vi "projekt.vi"() -> ()   [LabVIEW 2023]
doc: "Use this template to build a standard state machine design pattern. Each state executes code and determines which state to transition to. Contrast this design pattern with the User Interface Event Handler pattern, in which code executes in response to user actions. Contrast this design pattern also with the Queued Message Handler pattern, in which each message handling code can queue zero or more new messages.\nNote: This template does not contain the most recent programming guidelines recommended by National Instruments. For a complete, project-based implementation of the Standard State Machine pattern, use the Create Project dialog box instead of this template."
uses:
  projekt_stany.ctl
  <vilib>/DAQmx/read.llb/DAQmx Read (Digital 1D Bool 1Chan 1Samp).vi
  <vilib>/DAQmx/create/channels.llb/DAQmx Create Channel (DI-Digital Input).vi
  <vilib>/DAQmx/miscellaneous.llb/DAQmx Fill In Error Info.vi
panel:
  in  "Wyczysc":bool
  out "String 9":string
  out "String 8":string
  out "String 7":string
  out "String 6":string
  out "String 5":string
  out "String 4":string
  out "String 3":string
  out "String 2":string
  out "String":string
  out "Nastepny Gracz":string
  in  "Wybierz Kto zaczyna":bool
  out "Wynik":string
  in  "Stop":bool
  out "Kolumna":dbl
  out "Wiersz":dbl
  # "INSTRUKCJA GRY:"
  # "Aby wyczysc plansze, nalezy kliknac przycisk WYCZYSC na panelu glownym\noraz zatwierdzic CZERWONYM przyciskiem."
  # "Mozna wybrac kolejnosc czy O ma byc pierwsze czy moze X:\n - Jezeli przycisk jest wlaczony to zaczyna gracz X\n - Jezeli przycisk jest wylaczony to zaczyna gracz O\n\nJednak kolejnosc musi byc wybrana przed zaczeciem gry."
  # "Aby wybrac pole w którym ma byc wstawiony symbol nalezy wybrac kolumne oraz wiersz  (1 - 3) uzywajac przyciskow na urzadzeniu, aby dowiedziec sie za co opowiadaja przyciski przejdz do sekcji \"INSTRUKCJA DO PRZYCISKÓW\""
  # "INSTRUKCJA DO PRZYCISKÓW:"
  # "- Do wyboru wiersza sluzy przycisk ZIELONY\n - Do wyboru kolumny sluzy przycisk NIEBIESKI\n - Do zatwierdzenia swojego wyboru sluzy przycisk CZERWONY"
  # "SCHEMAT WYBORU POLA:"
  # "SCIAGAWKA PRZY WYBIERANIU POLA:"
  # "[ WIERSZ, KOLUMNA ]"
  # "[ 1, 1 ]  [ 1, 2 ]  [ 1, 3 ]\n[ 2, 1 ]  [ 2, 2 ]  [ 2, 3 ]\n[ 3, 1 ]  [ 3, 2 ]  [ 3, 3 ]"
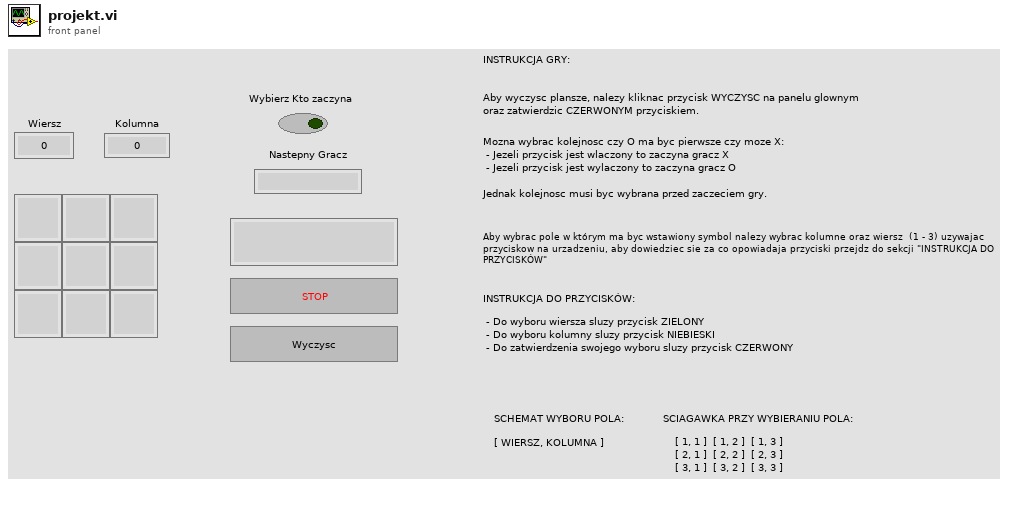
[diagram p1: front panel]
types:
  T1 = typedef "projekt_stany.ctl" = enum16{"Czysc", "Zapisz", "Wpisz", "Sprawdz", "Czytaj", "Initialize", "Stop"}
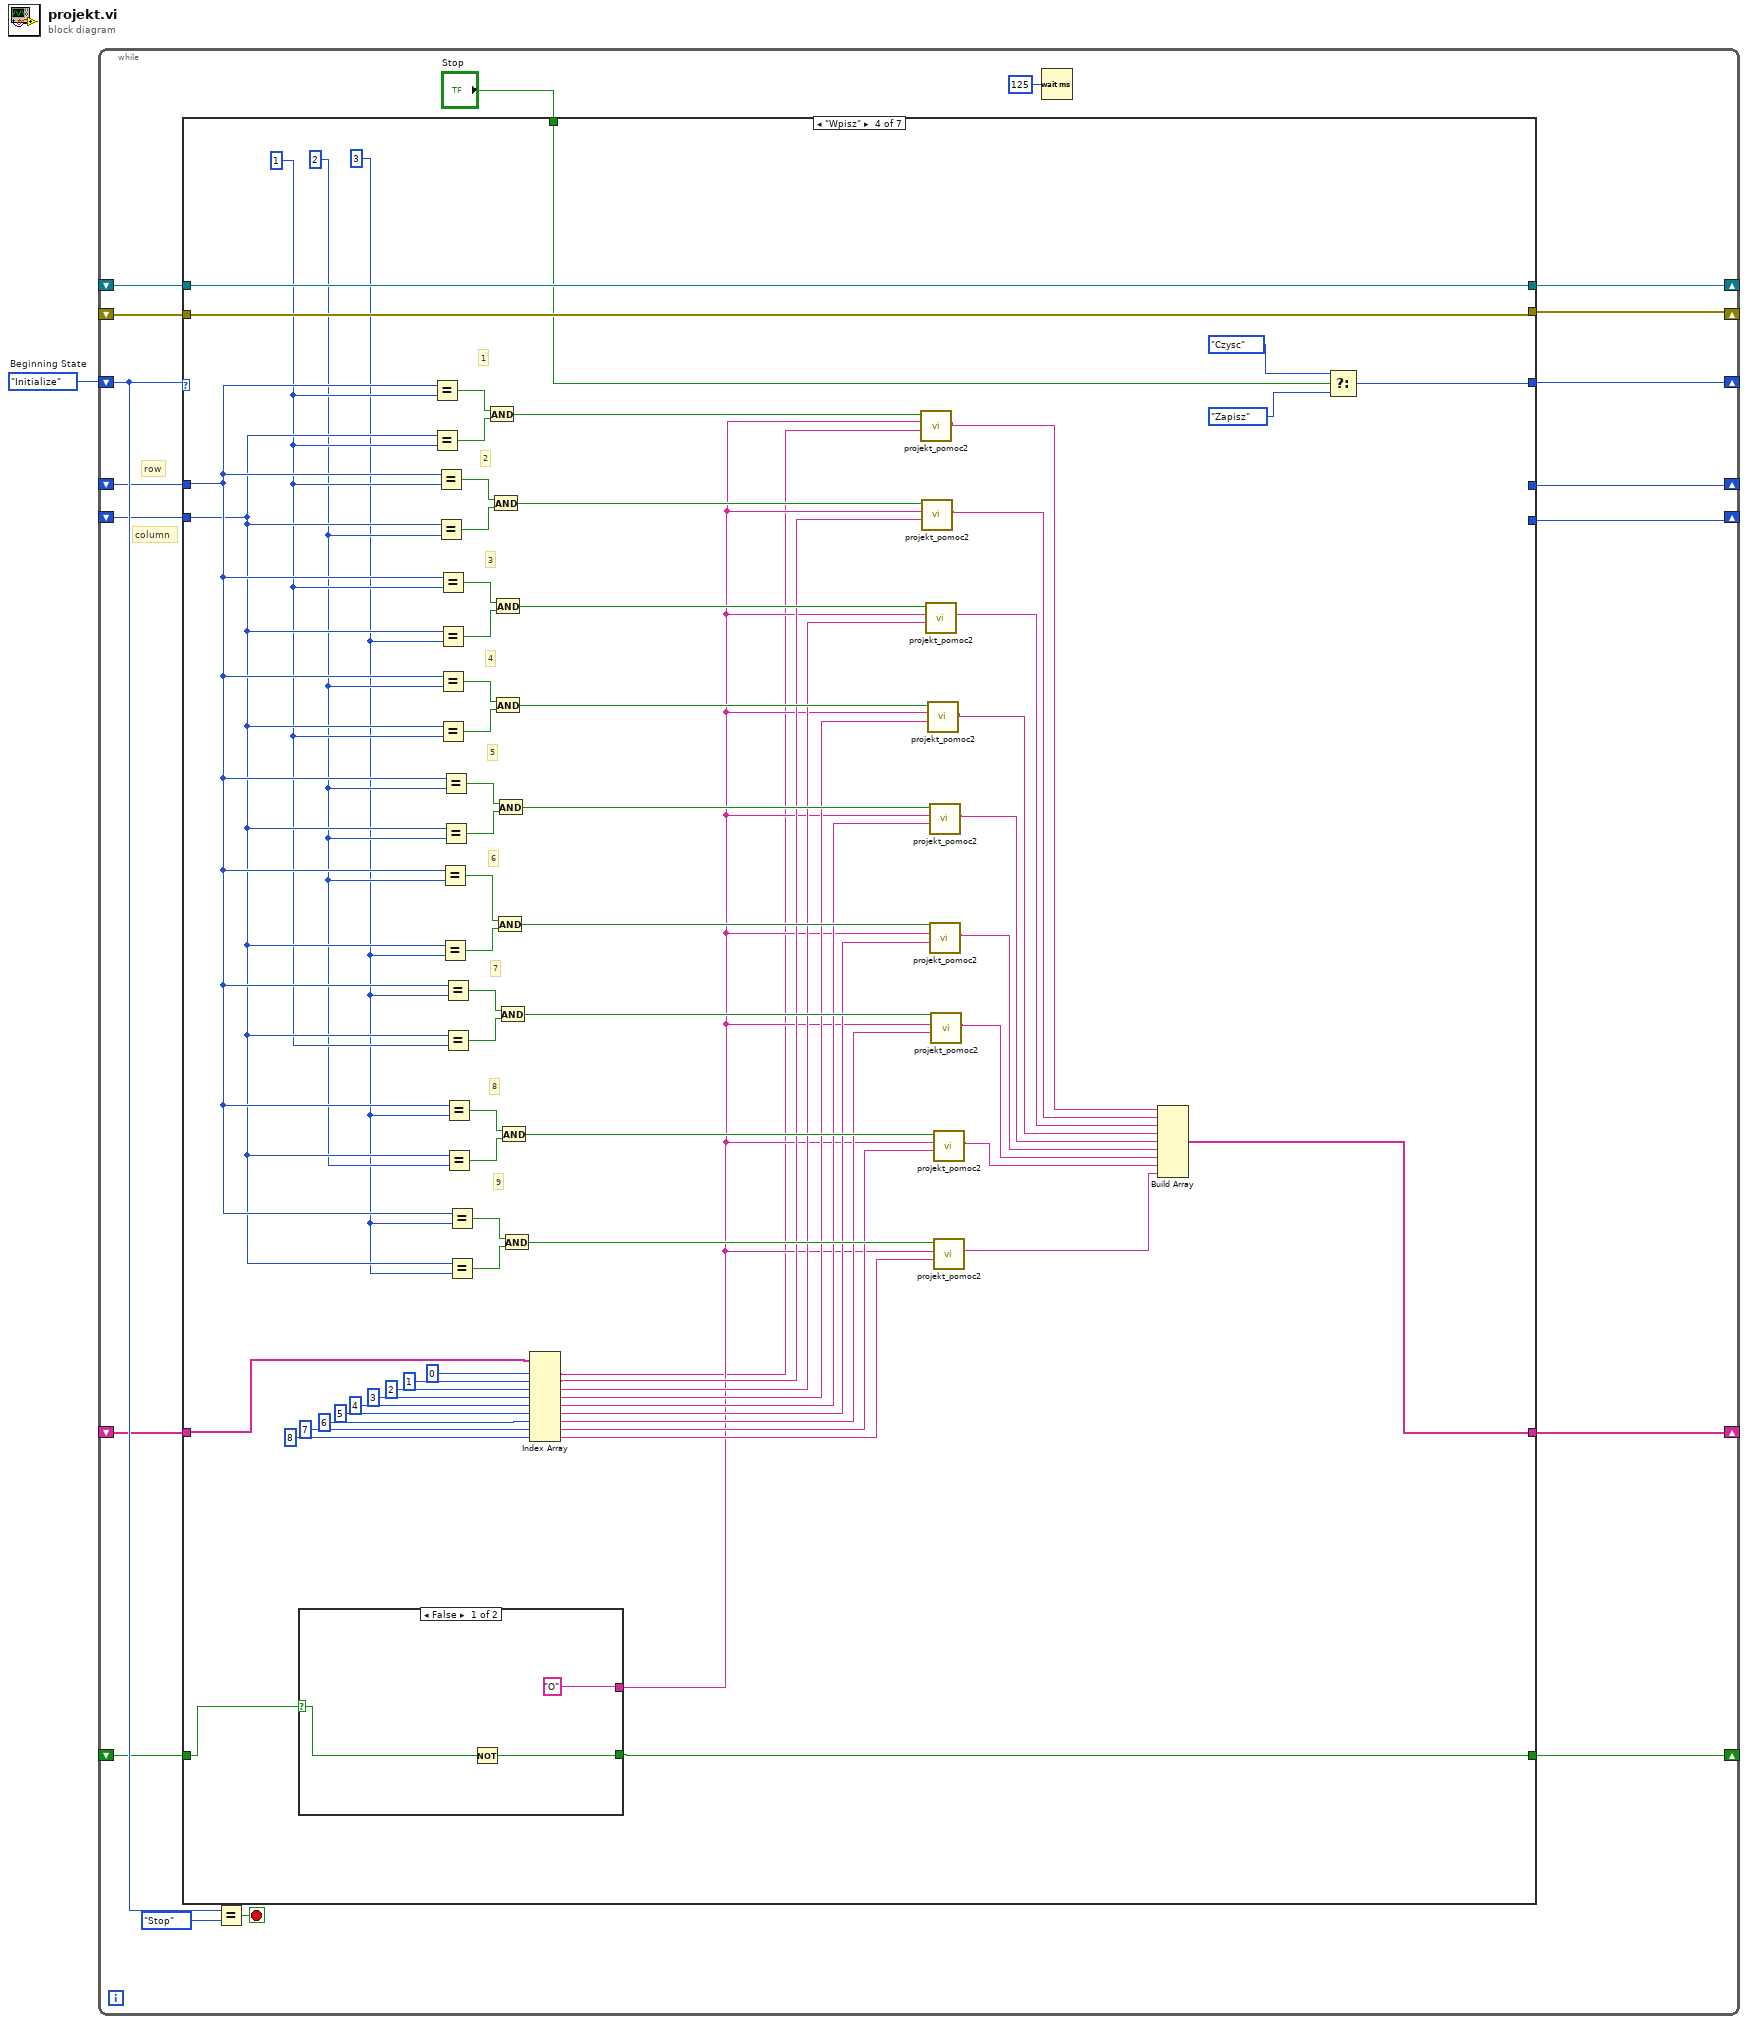
[diagram p0: block diagram]
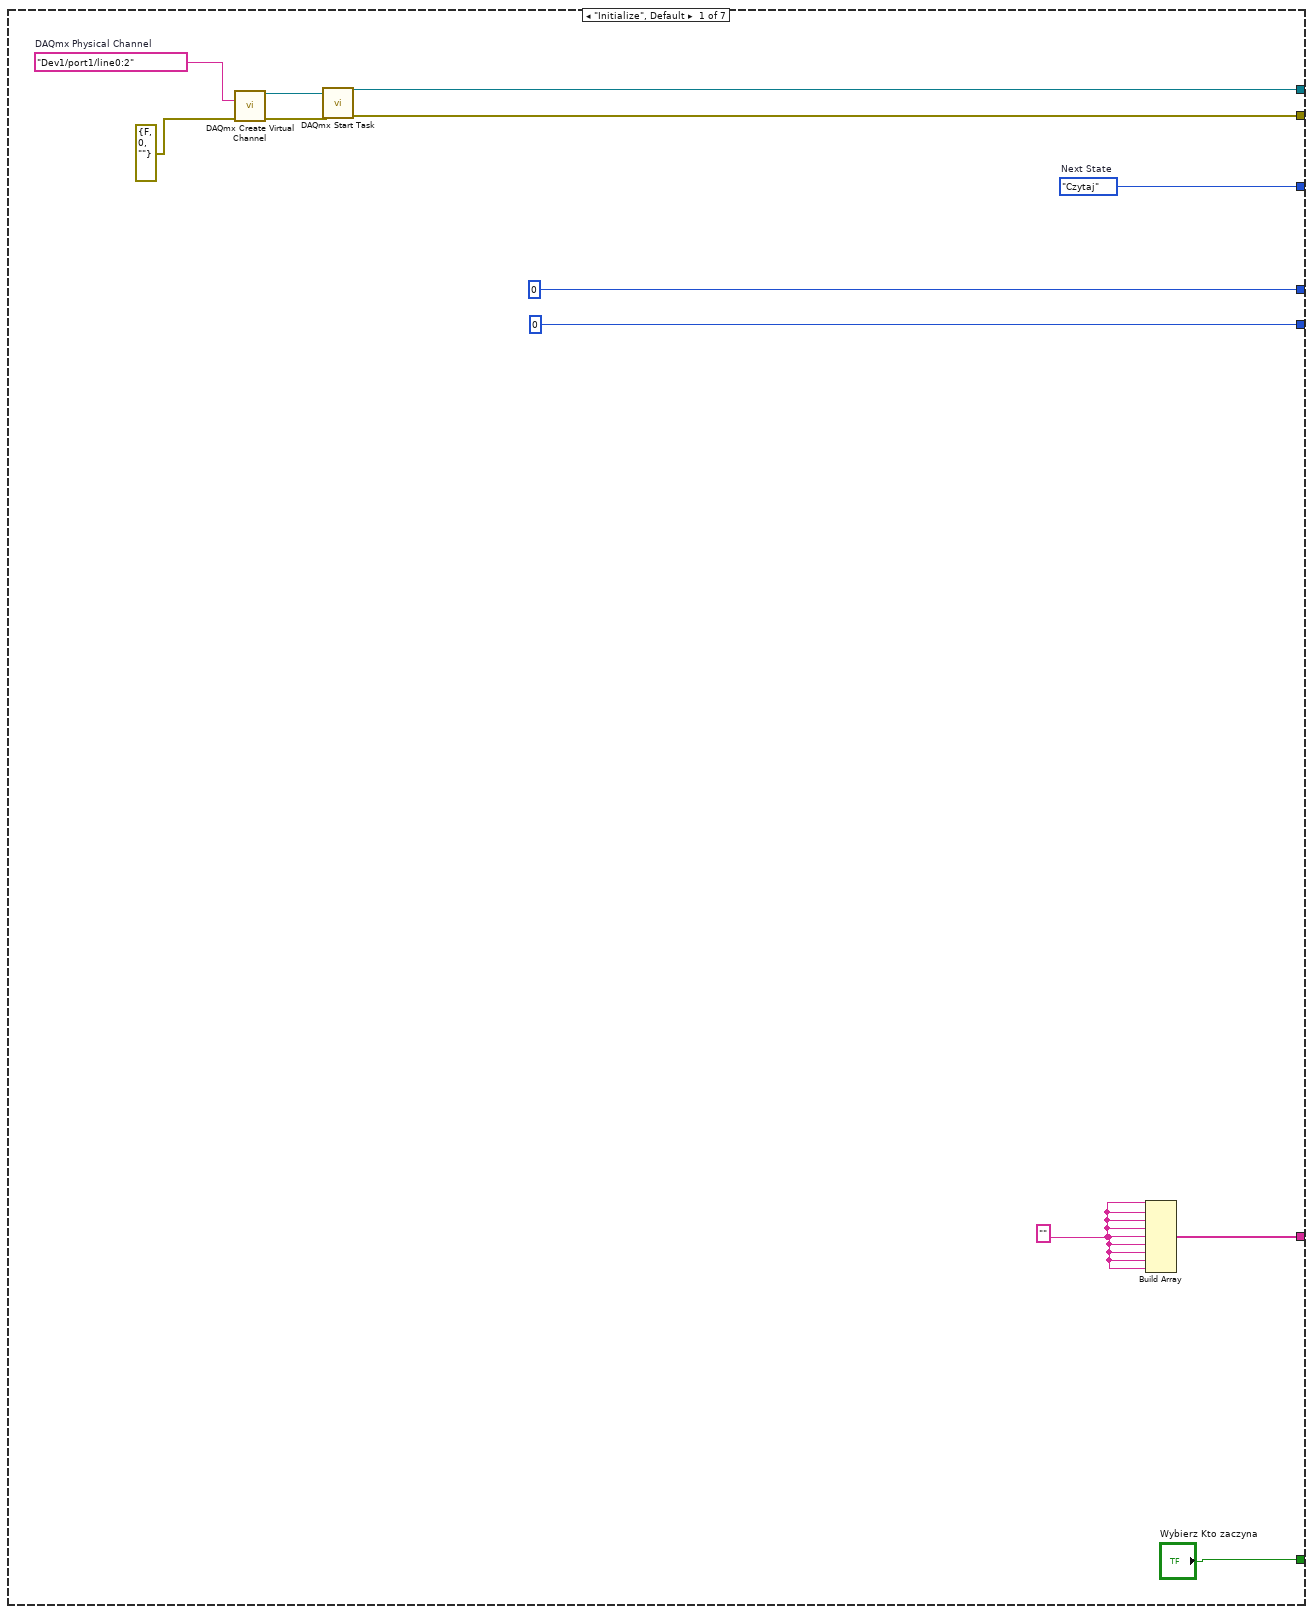
[diagram p2: hidden frame]
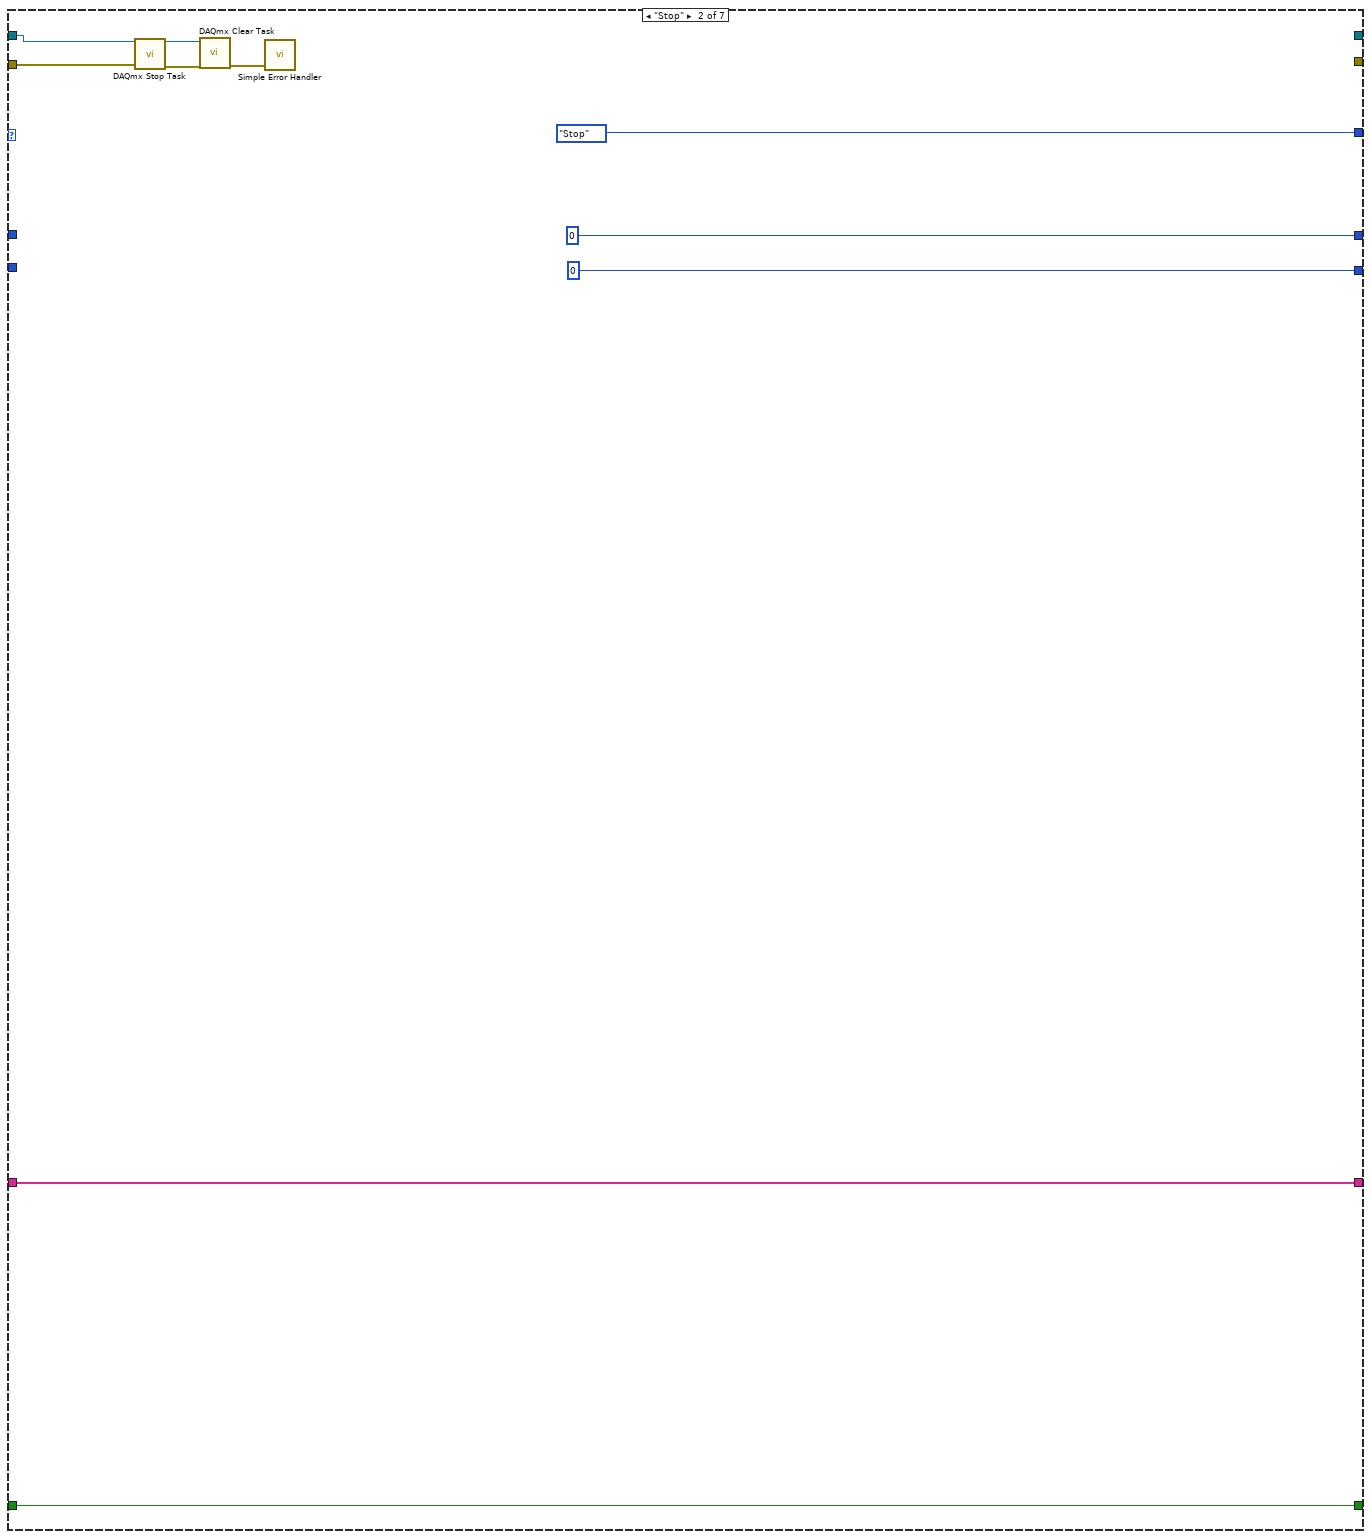
[diagram p3: hidden frame]
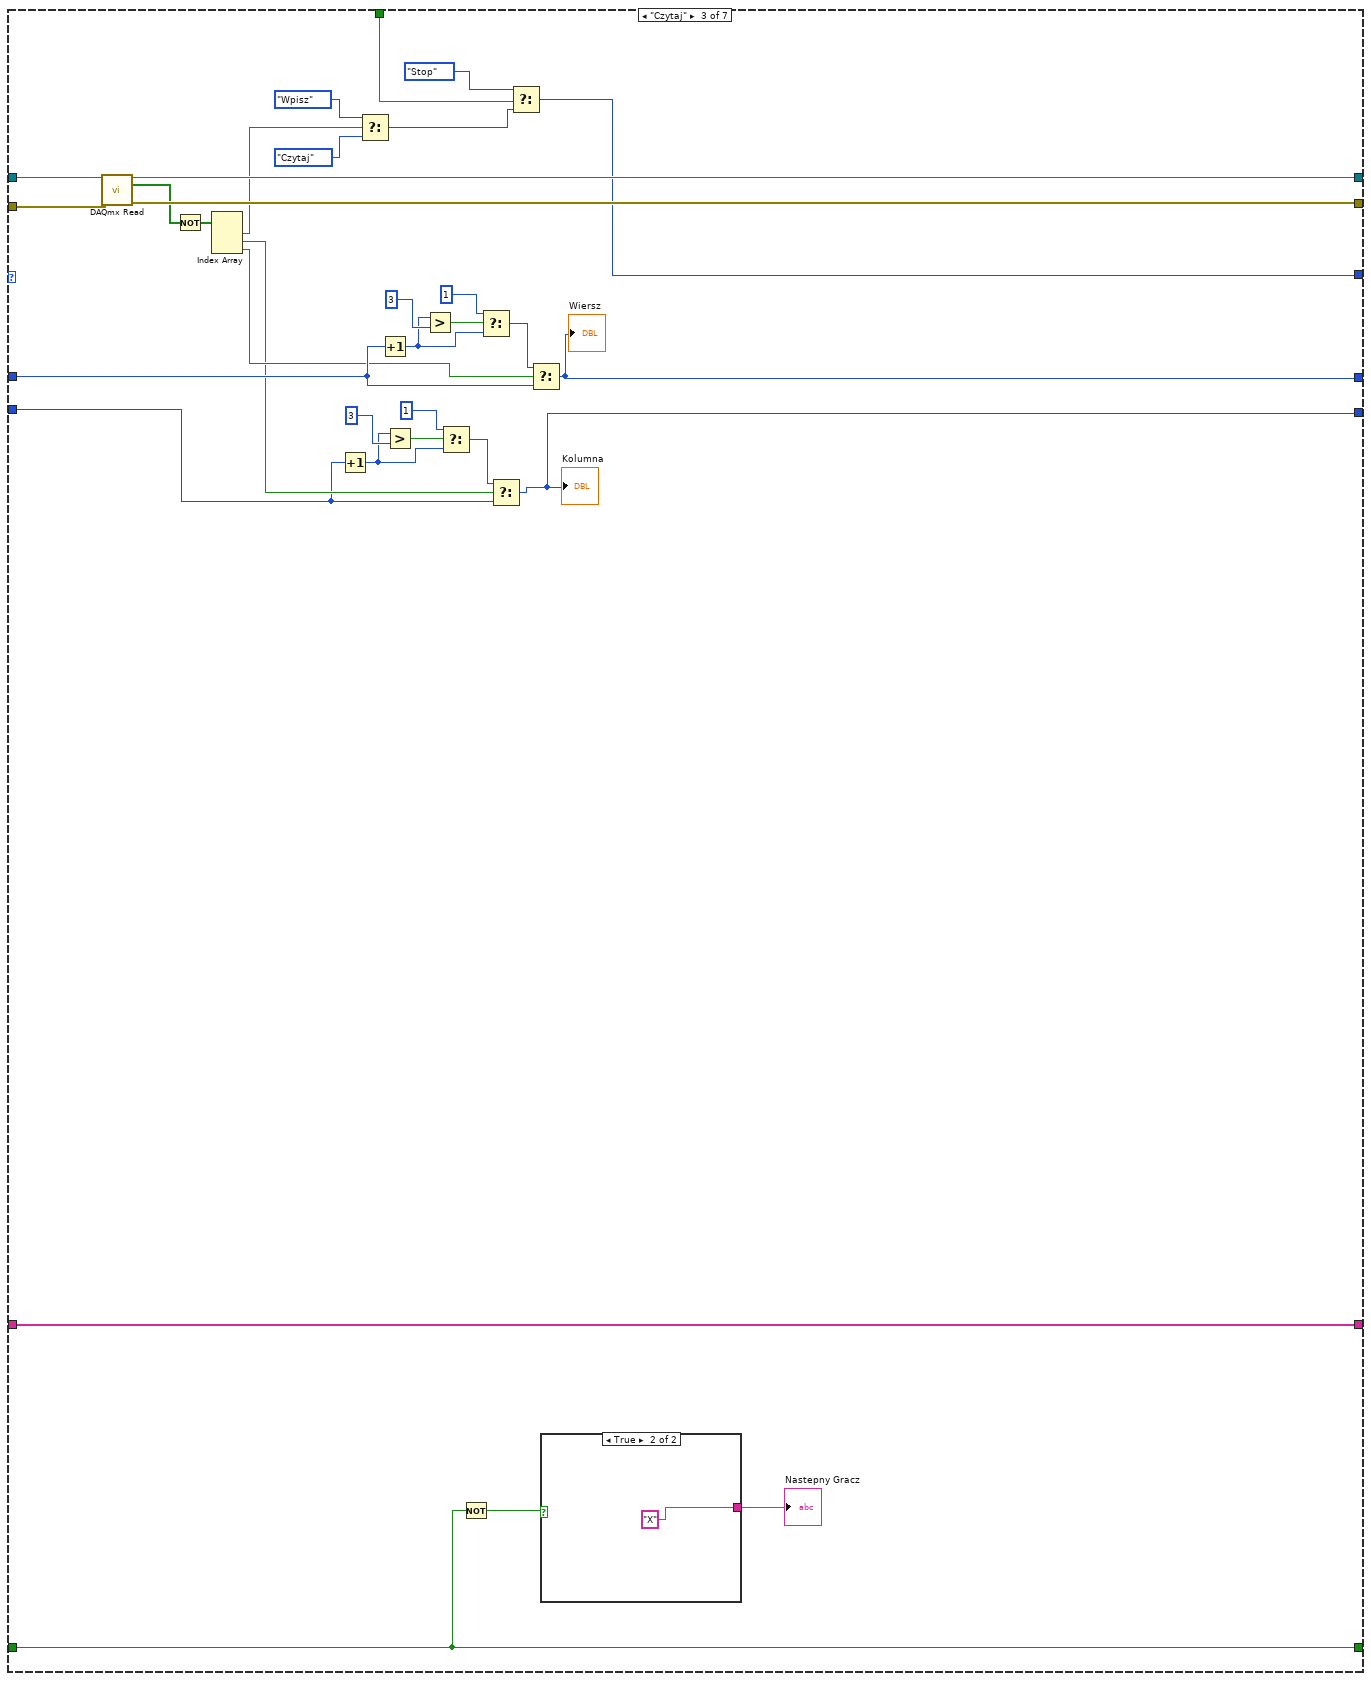
[diagram p4: hidden frame]
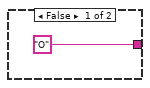
[diagram p5: hidden frame]
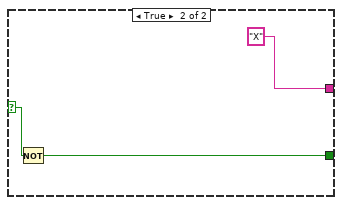
[diagram p6: hidden frame]
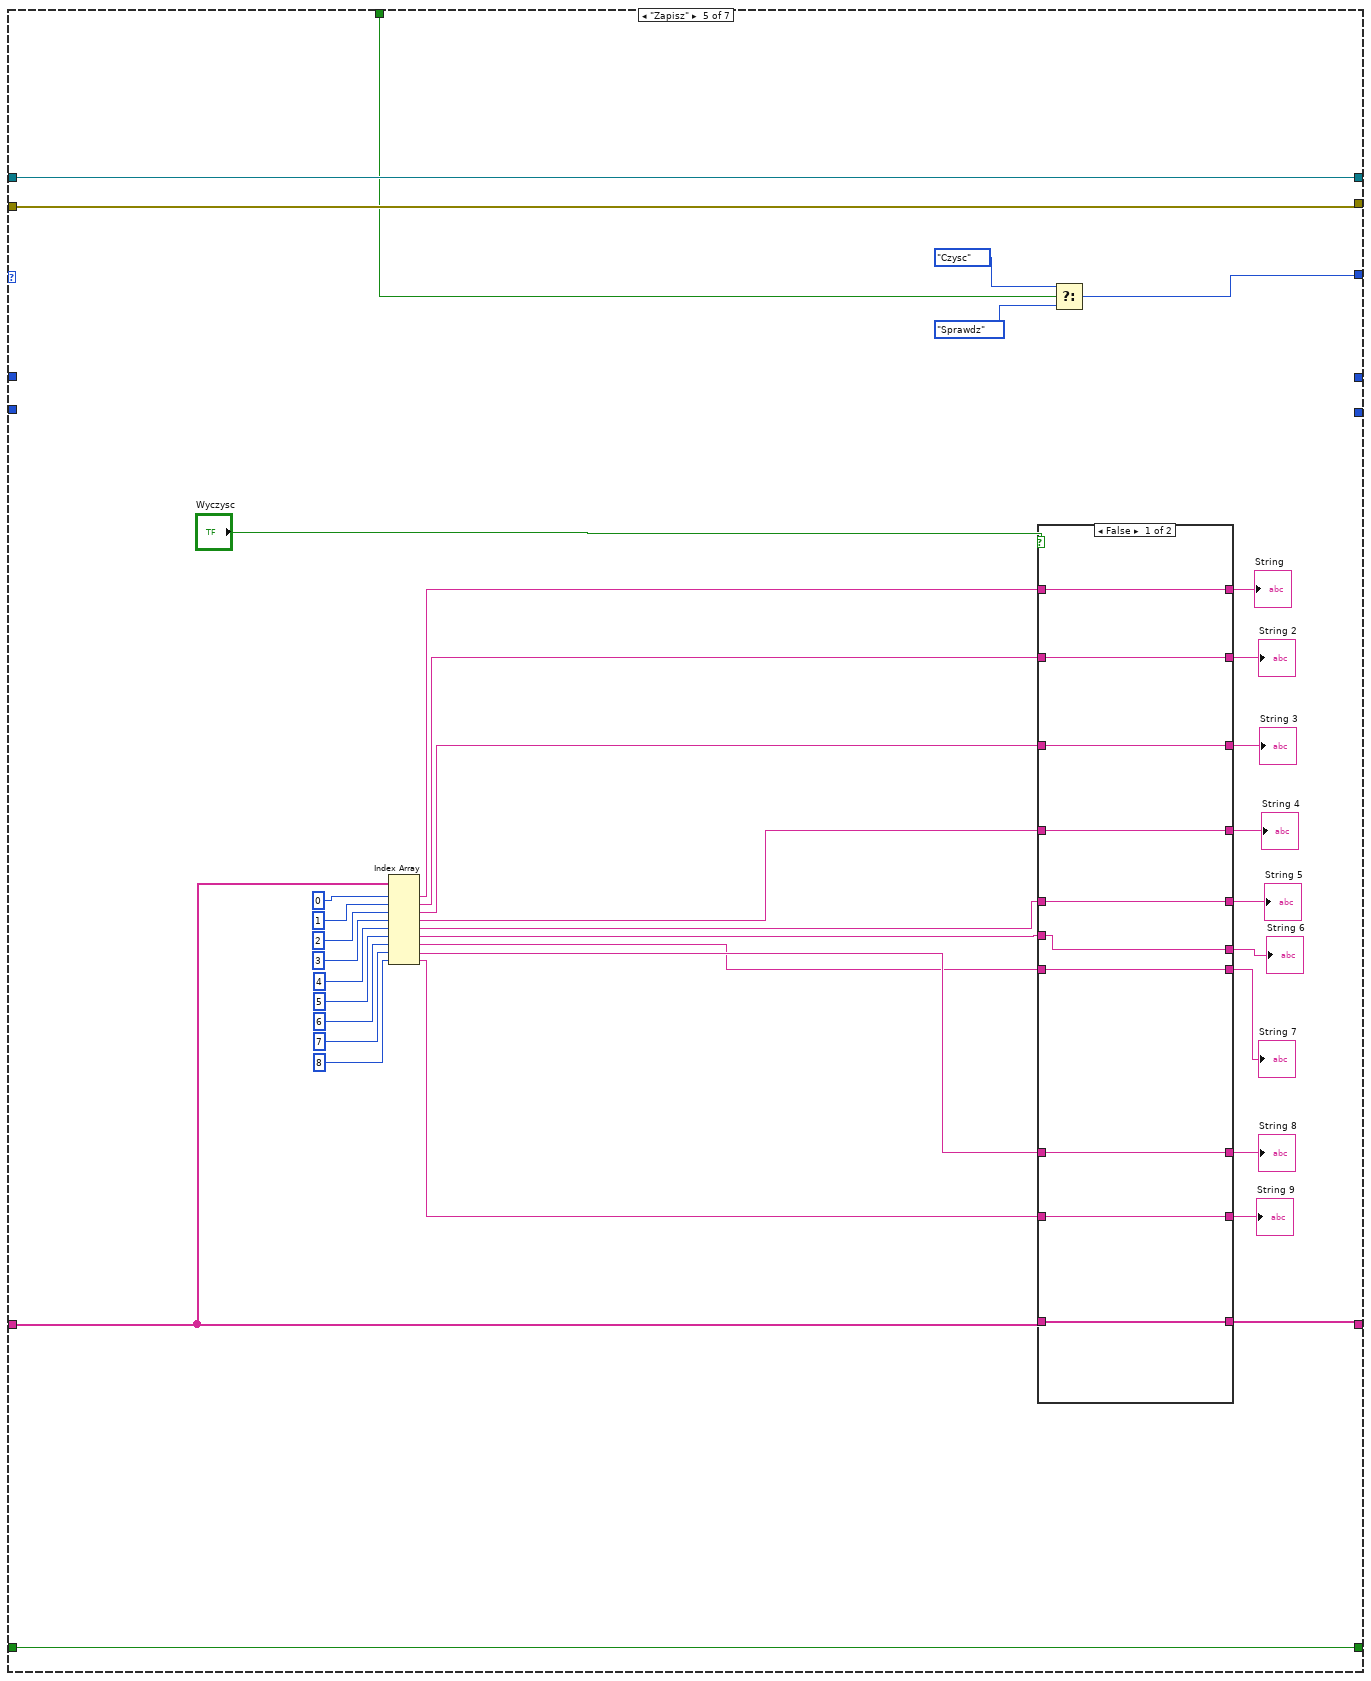
[diagram p7: hidden frame]
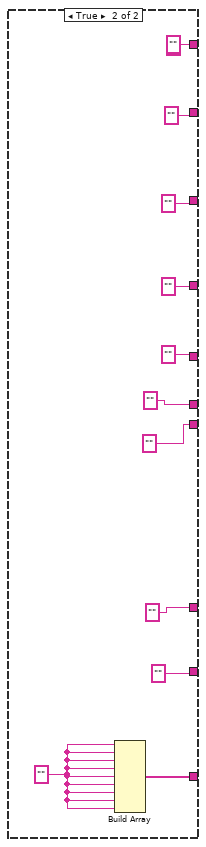
[diagram p8: hidden frame]
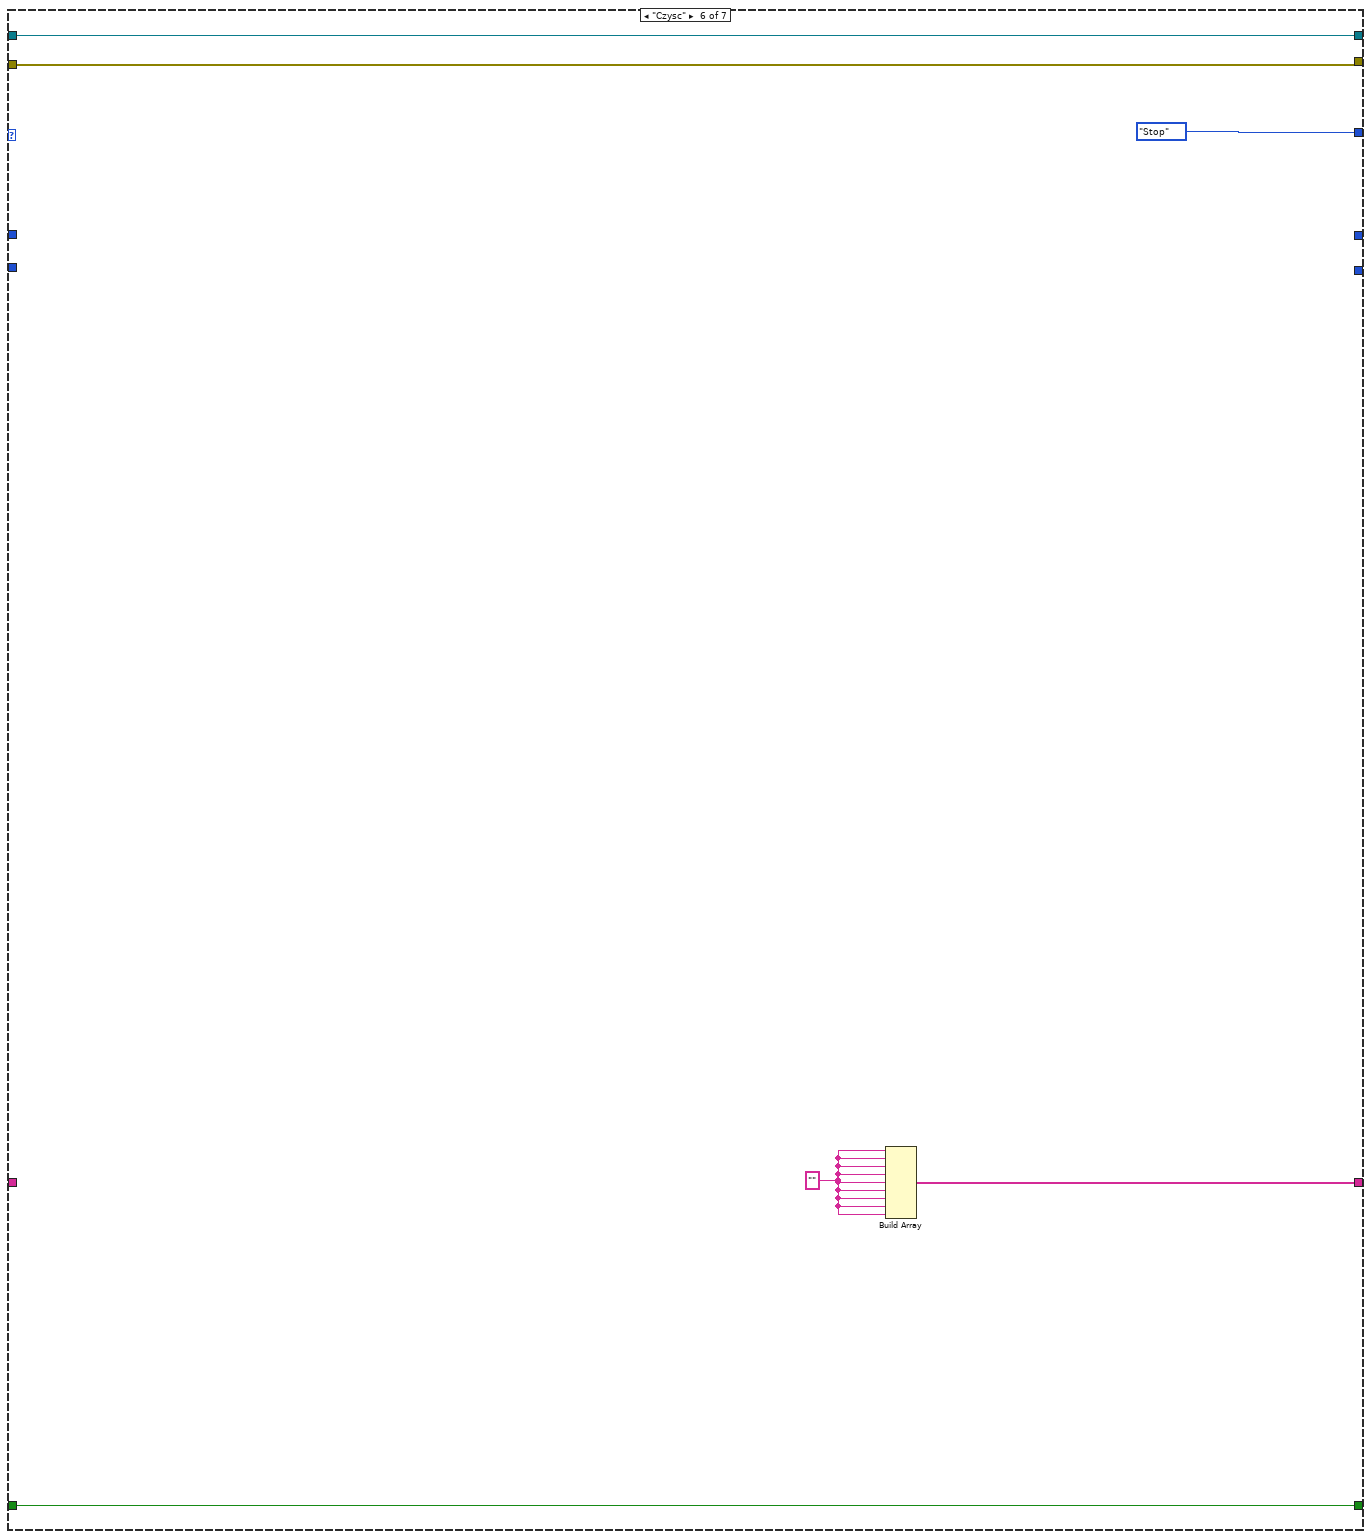
[diagram p9: hidden frame]
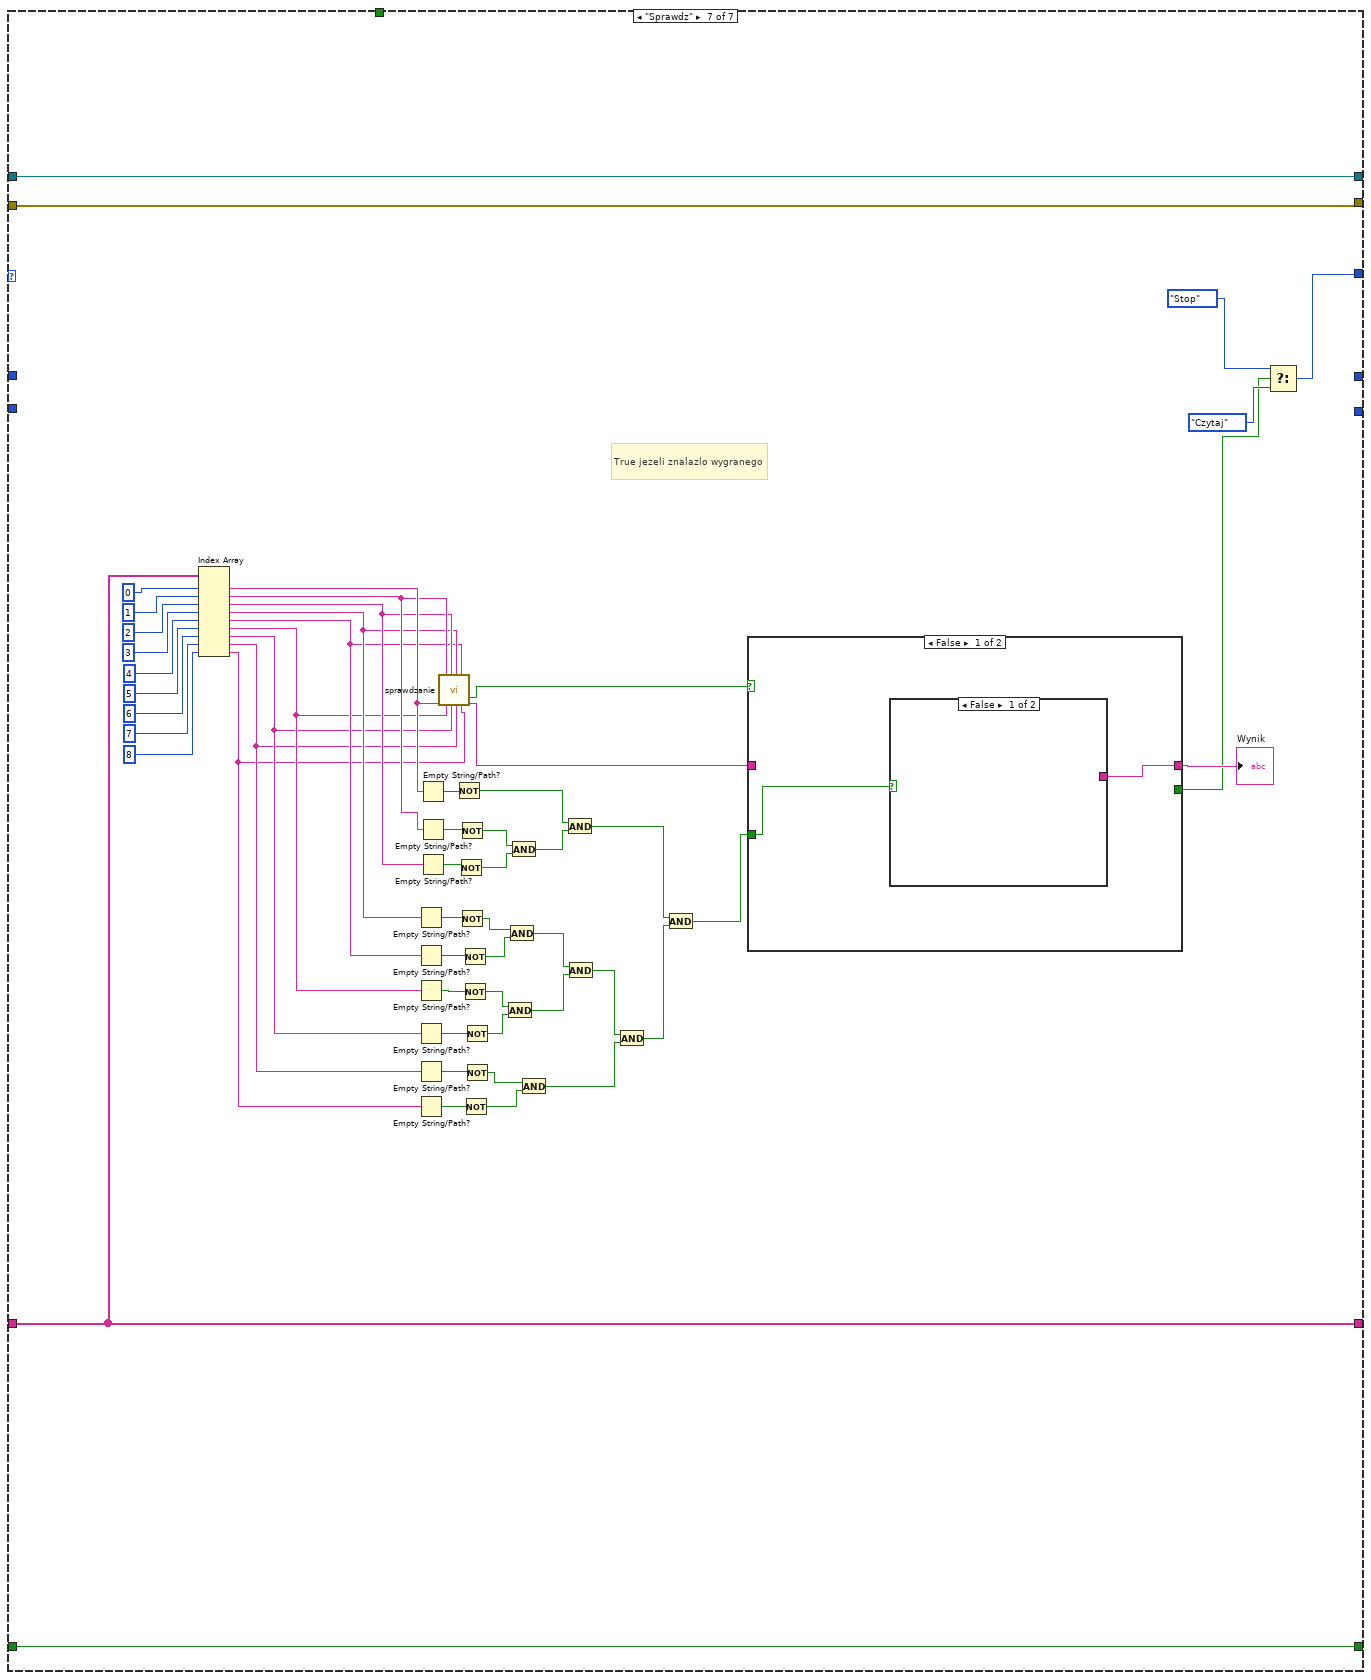
[diagram p10: hidden frame]
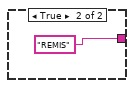
[diagram p11: hidden frame]
diagram:
  w1 = projekt_stany."Initialize"  # Beginning State
  n1 = while {
    shift-right: [w16] -> _
    shift-left: w1 -> [w17]
    shift-right: [w14] -> _
    shift-left: _ -> [w12]
    shift-right: [w13] -> _
    shift-left: _ -> [w11]
    shift-right: [w10] -> _
    shift-left: _ -> [w7]
    shift-right: [w9] -> _
    shift-left: _ -> [w8]
    shift-right: [w5] -> _
    shift-left: _ -> [w4]
    shift-right: [w2] -> _
    shift-left: _ -> [w3]
    stop <- w19 stop-if-true
    # "column"
    # "row"
    n2 = case shown="\"Wpisz\"" w17 {
      tunnel: [w20 projekt_stany."Stop" ("Next State") w47 w119 w184 projekt_stany."Stop" ("Next State") w257] -> w16
      tunnel: [w27 _ w72 w145 w188 w215 w270] -> w14
      tunnel: [w26 _ w71 w146 w189 w216 w271] -> w13
      tunnel: w12 -> [_ w39 w74 w145 w188 w215 w270]
      tunnel: w11 -> [_ w40 w73 w146 w189 w216 w271]
      tunnel: [0 0 w69 _ _ _ _] -> w10
      tunnel: [0 0 w55 _ _ _ _] -> w9
      tunnel: w8 -> [_ _ w53 w125 _ _ _]
      tunnel: w7 -> [_ _ w70 w126 _ _ _]
      tunnel: "Stop" -> [_ _ w46 w77 w183 _ _]
      tunnel: ["Wybierz Kto zaczyna" w33 w43 w107 w187 w214 w260] -> w5
      tunnel: w4 -> [_ w33 w43 w118 w187 w214 w260]
      tunnel: w3 -> [_ w32 w45 w104 w153 _ w256]
      tunnel: [w22 w32 w45 w108 w154 w212 w256] -> w2
      frame "Initialize", Default {
        w20 = projekt_stany."Czytaj"  # Next State
        w23 = ""
        w28 = tag "Dev1/port1/line0:2"  # DAQmx Physical Channel
        n3 = call-poly <vilib>:"DAQmx Create Virtual Channel.vi"("lines"=w28, "error in"=errorcluster {"status"=FALSE, "code"=0, "source"=""} ("error constant")) -> ("task out"=w29:refnum<k21>, "error out"=w30:errorcluster)  [unwired: 12 in]
        n4 = call <vilib>:"DAQmx Start Task.vi"("task/channels in"=w29, "error in"=w30) -> ("task out"=w26:refnum<k21>, "error out"=w27:errorcluster)  [unwired: 12 in]
        n5 = Build Array(w23, w23, w23, w23, w23, w23, w23, w23, w23) -> (w22:string[])
      }
      frame "Stop" {
        n6 = call <vilib>:"DAQmx Stop Task.vi"("task/channels in"=w40, "error in"=w39) -> ("task out"=w38:refnum<k21>, "error out"=w37:errorcluster)  [unwired: 12 in]
        n7 = call <vilib>:"DAQmx Clear Task.vi"("task in"=w38, "error in"=w37) -> ("error out"=w36:errorcluster)  [unwired: 13 in]
        n8 = call <vilib>:"Simple Error Handler.vi"("error in (no error)"=w36) -> ()  [unwired: 4 in, 5 out]
      }
      frame "Czytaj" {
        n9 = call-poly <vilib>:"DAQmx Read.vi"("task/channels in"=w73, "error in"=w74) -> ("task out"=w71:refnum<k21>, "data"=w63:bool[], "error out"=w72:errorcluster)  [unwired: 11 in]
        n10 = Not(x=w63) -> (.not. x?=w62:bool[])
        n11 = Index Array(array=w62) -> (element #1=w52:bool, element #2=w54:bool, element #3=w61:bool)  [unwired: 3 in]
        n12 = Increment(x=w53) -> (x+1=w57:i32)
        n13 = Select(t=projekt_stany."Wpisz" ("Next State"), s=w52, f=projekt_stany."Czytaj" ("Next State")) -> (s? t:f=w49:T1)
        n14 = Increment(x=w70) -> (x+1=w65:i32)
        n15 = Greater?(x=w57, y=3) -> (0:w59:bool)
        n16 = Greater?(x=w65, y=3) -> (0:w67:bool)
        n17 = Select(t=1, s=w59, f=w57) -> (s? t:f=w56:i32)
        n18 = Not(x=w43) -> (.not. x?=w44:bool)
        n19 = Select(t=1, s=w67, f=w65) -> (s? t:f=w64:i32)
        n20 = Select(t=w56, s=w54, f=w53) -> (s? t:f=w55:i32)
        "Kolumna" <- w55
        n21 = Select(t=projekt_stany."Stop" ("Next State"), s=w46, f=w49) -> (s? t:f=w47:T1)
        n22 = Select(t=w64, s=w61, f=w70) -> (s? t:f=w69:i32)
        "Wiersz" <- w69
        n23 = case shown="True" w44 {
          tunnel: ["O" "X"] -> w42
          frame False {
          }
          frame True {
          }
        }
        "Nastepny Gracz" <- w42
      }
      frame "Wpisz" {
        w122 = 3
        w123 = 2
        w124 = 1
        # "9"
        # "8"
        # "7"
        # "6"
        # "5"
        # "4"
        # "3"
        # "2"
        # "1"
        n24 = case shown="False" w118 {
          selector: w118 -> [w148 w151]
          tunnel: ["O" "X"] -> w80
          tunnel: [w147 w150] -> w107
          frame False {
            n25 = Not(x=w148) -> (.not. x?=w147:bool)
          }
          frame True {
            n26 = Not(x=w151) -> (.not. x?=w150:bool)
          }
        }
        n27 = Equal?(x=w126, y=w124) -> (x = y?=w144:bool)
        n28 = Equal?(x=w125, y=w124) -> (x = y?=w143:bool)
        n29 = Equal?(x=w126, y=w124) -> (x = y?=w142:bool)
        n30 = Equal?(x=w125, y=w123) -> (x = y?=w141:bool)
        n31 = Equal?(x=w126, y=w124) -> (x = y?=w140:bool)
        n32 = Equal?(x=w125, y=w122) -> (x = y?=w139:bool)
        n33 = Equal?(x=w126, y=w123) -> (x = y?=w138:bool)
        n34 = Equal?(x=w125, y=w124) -> (x = y?=w137:bool)
        n35 = Equal?(x=w126, y=w123) -> (x = y?=w134:bool)
        n36 = Equal?(x=w125, y=w122) -> (x = y?=w133:bool)
        n37 = Equal?(x=w126, y=w123) -> (x = y?=w136:bool)
        n38 = Equal?(x=w125, y=w123) -> (x = y?=w135:bool)
        n39 = Equal?(x=w126, y=w122) -> (x = y?=w132:bool)
        n40 = Equal?(x=w125, y=w124) -> (x = y?=w131:bool)
        n41 = Equal?(x=w126, y=w122) -> (x = y?=w130:bool)
        n42 = Equal?(x=w125, y=w123) -> (x = y?=w129:bool)
        n43 = Equal?(x=w126, y=w122) -> (x = y?=w128:bool)
        n44 = Equal?(x=w125, y=w122) -> (x = y?=w127:bool)
        n45 = And(x=w144, y=w143) -> (x .and. y?=w81:bool)
        n46 = And(x=w142, y=w141) -> (x .and. y?=w84:bool)
        n47 = And(x=w140, y=w139) -> (x .and. y?=w87:bool)
        n48 = And(x=w138, y=w137) -> (x .and. y?=w90:bool)
        n49 = And(x=w134, y=w133) -> (x .and. y?=w96:bool)
        n50 = And(x=w136, y=w135) -> (x .and. y?=w93:bool)
        n51 = And(x=w132, y=w131) -> (x .and. y?=w99:bool)
        n52 = And(x=w130, y=w129) -> (x .and. y?=w102:bool)
        n53 = And(x=w128, y=w127) -> (x .and. y?=w105:bool)
        n54 = Index Array(array=w104, index #1=0, index #2=1, index #3=2, index #4=3, index #5=4, index #6=5, index #7=6, index #8=7, index #9=8) -> (element #1=w79:string, element #2=w83:string, element #3=w86:string, element #4=w89:string, element #5=w92:string, element #6=w95:string, element #7=w98:string, element #8=w101:string, element #9=w103:string)
        n55 = call "projekt_pomoc2.vi"("String 2"=w79, "String"=w80, "Boolean"=w81) -> ("String 3"=w78:string)  [unwired: 8 in]
        n56 = call "projekt_pomoc2.vi"("String 2"=w83, "String"=w80, "Boolean"=w84) -> ("String 3"=w82:string)  [unwired: 8 in]
        n57 = call "projekt_pomoc2.vi"("String 2"=w86, "String"=w80, "Boolean"=w87) -> ("String 3"=w85:string)  [unwired: 8 in]
        n58 = call "projekt_pomoc2.vi"("String 2"=w89, "String"=w80, "Boolean"=w90) -> ("String 3"=w88:string)  [unwired: 8 in]
        n59 = call "projekt_pomoc2.vi"("String 2"=w92, "String"=w80, "Boolean"=w93) -> ("String 3"=w91:string)  [unwired: 8 in]
        n60 = call "projekt_pomoc2.vi"("String 2"=w95, "String"=w80, "Boolean"=w96) -> ("String 3"=w94:string)  [unwired: 8 in]
        n61 = call "projekt_pomoc2.vi"("String 2"=w98, "String"=w80, "Boolean"=w99) -> ("String 3"=w97:string)  [unwired: 8 in]
        n62 = call "projekt_pomoc2.vi"("String 2"=w101, "String"=w80, "Boolean"=w102) -> ("String 3"=w100:string)  [unwired: 8 in]
        n63 = call "projekt_pomoc2.vi"("String 2"=w103, "String"=w80, "Boolean"=w105) -> ("String 3"=w106:string)  [unwired: 8 in]
        n64 = Build Array(w78, w82, w85, w88, w91, w94, w97, w100, w106) -> (w108:string[])
        n65 = Select(t=projekt_stany."Czysc" ("Next State"), s=w77, f=projekt_stany."Zapisz" ("Next State")) -> (s? t:f=w119:T1)
      }
      frame "Zapisz" {
        n66 = Index Array(array=w153, index #1=0, index #2=1, index #3=2, index #4=3, index #5=4, index #6=5, index #7=6, index #8=7, index #9=8) -> (element #1=w164:string, element #2=w165:string, element #3=w166:string, element #4=w167:string, element #5=w168:string, element #6=w169:string, element #7=w170:string, element #8=w171:string, element #9=w172:string)
        n67 = case shown="False" "Wyczysc" {
          tunnel: w172 -> [w191 _]
          tunnel: w171 -> [w192 _]
          tunnel: w170 -> [w194 _]
          tunnel: w169 -> [w193 _]
          tunnel: w168 -> [w195 _]
          tunnel: w167 -> [w196 _]
          tunnel: w166 -> [w197 _]
          tunnel: w165 -> [w198 _]
          tunnel: w164 -> [w199 _]
          tunnel: [w199 ""] -> w163
          tunnel: [w198 ""] -> w162
          tunnel: [w197 ""] -> w161
          tunnel: [w196 ""] -> w160
          tunnel: [w195 ""] -> w159
          tunnel: [w193 ""] -> w158
          tunnel: [w194 ""] -> w157
          tunnel: [w192 ""] -> w156
          tunnel: [w191 ""] -> w155
          tunnel: [w190 w200] -> w154
          tunnel: w153 -> [w190 _]
          frame False {
          }
          frame True {
            w201 = ""
            (unwired) ""
            n68 = Build Array(w201, w201, w201, w201, w201, w201, w201, w201, w201) -> (w200:string[])
          }
        }
        "String" <- w163
        "String 2" <- w162
        "String 3" <- w161
        "String 4" <- w160
        "String 5" <- w159
        "String 6" <- w158
        "String 7" <- w157
        "String 8" <- w156
        "String 9" <- w155
        n69 = Select(t=projekt_stany."Czysc" ("Next State"), s=w183, f=projekt_stany."Sprawdz" ("Next State")) -> (s? t:f=w184:T1)
      }
      frame "Czysc" {
        w213 = ""
        n70 = Build Array(w213, w213, w213, w213, w213, w213, w213, w213, w213) -> (w212:string[])
      }
      frame "Sprawdz" {
        # "True jezeli znalazlo wygranego"
        n71 = Index Array(array=w256, index #1=0, index #2=1, index #3=2, index #4=3, index #5=4, index #6=5, index #7=6, index #8=7, index #9=8) -> (element #1=w227:string, element #2=w226:string, element #3=w225:string, element #4=w224:string, element #5=w223:string, element #6=w220:string, element #7=w219:string, element #8=w218:string, element #9=w217:string)
        n72 = Empty String/Path?(string/path=w224) -> (empty?=w250:bool)
        n73 = Empty String/Path?(string/path=w223) -> (empty?=w251:bool)
        n74 = Empty String/Path?(string/path=w220) -> (empty?=w252:bool)
        n75 = Empty String/Path?(string/path=w219) -> (empty?=w253:bool)
        n76 = Empty String/Path?(string/path=w218) -> (empty?=w254:bool)
        n77 = Empty String/Path?(string/path=w217) -> (empty?=w255:bool)
        n78 = Empty String/Path?(string/path=w227) -> (empty?=w247:bool)
        n79 = Empty String/Path?(string/path=w226) -> (empty?=w248:bool)
        n80 = Empty String/Path?(string/path=w225) -> (empty?=w249:bool)
        n81 = call "sprawdzanie.vi"("String"=w227, "String 2"=w226, "String 6"=w220, "String 3"=w225, "String 7"=w219, "String 4"=w224, "String 8"=w218, "String 5"=w223, "String 9"=w217) -> ("X or O"=w221:bool, "String 10"=w222:string)  [unwired: 9 in]
        n82 = Not(x=w247) -> (.not. x?=w238:bool)
        n83 = Not(x=w249) -> (.not. x?=w240:bool)
        n84 = Not(x=w248) -> (.not. x?=w239:bool)
        n85 = Not(x=w250) -> (.not. x?=w241:bool)
        n86 = Not(x=w251) -> (.not. x?=w242:bool)
        n87 = Not(x=w252) -> (.not. x?=w243:bool)
        n88 = Not(x=w255) -> (.not. x?=w246:bool)
        n89 = Not(x=w253) -> (.not. x?=w244:bool)
        n90 = Not(x=w254) -> (.not. x?=w245:bool)
        n91 = And(x=w243, y=w244) -> (x .and. y?=w236:bool)
        n92 = And(x=w241, y=w242) -> (x .and. y?=w235:bool)
        n93 = And(x=w239, y=w240) -> (x .and. y?=w237:bool)
        n94 = And(x=w245, y=w246) -> (x .and. y?=w234:bool)
        n95 = And(x=w238, y=w237) -> (x .and. y?=w231:bool)
        n96 = And(x=w235, y=w236) -> (x .and. y?=w233:bool)
        n97 = And(x=w233, y=w234) -> (x .and. y?=w232:bool)
        n98 = And(x=w231, y=w232) -> (x .and. y?=w229:bool)
        n99 = case shown="False" w221 {
          selector: w221 -> [_ w278]
          tunnel: w222 -> [_ w277]
          tunnel: [w272 w276] -> w230
          tunnel: w229 -> [w273 _]
          tunnel: [_ w275] -> w228
          frame False {
            n100 = case shown="False" w273 {
              tunnel: [_ "REMIS"] -> w272
              frame False {
              }
              frame True {
              }
            }
          }
          frame True {
            n101 = case shown="True" w278 {
              selector: w278 -> [_ w279]
              tunnel: w277 -> [_ w280]
              tunnel: [_ w280] -> w276
              tunnel: [_ w279] -> w275
              frame False {
              }
              frame True {
              }
            }
          }
        }
        "Wynik" <- w230
        n102 = Select(t=projekt_stany."Stop" ("Next State"), s=w228, f=projekt_stany."Czytaj" ("Next State")) -> (s? t:f=w257:T1)
      }
    }
    n103 = Equal?(x=w17, y=projekt_stany."Stop" ("States")) -> (x = y?=w19:bool)
    n104 = Wait (ms)(milliseconds to wait=u32 125) -> ()  [unwired: 1 out]
  }
